vi "使用 Navigation.vi"() -> ()   [LabVIEW 2018]
uses:
  Nagivation 2.0.lvclass
panel:
  out "二维图片":picture
  out "Distance":dbl
  in  "Destination In":cluster{"X":dbl, "Y":dbl}
  in  "Source In":cluster{"X":dbl, "Y":dbl}
  out "Source Out":cluster{"X":dbl, "Y":dbl}
  out "Destination Out":cluster{"X":dbl, "Y":dbl}
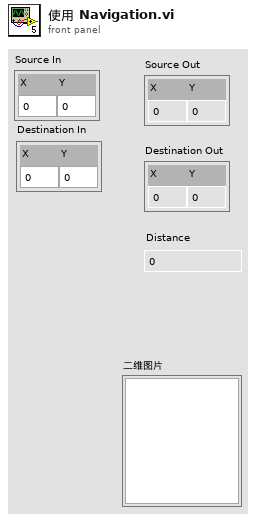
[diagram p1: front panel]
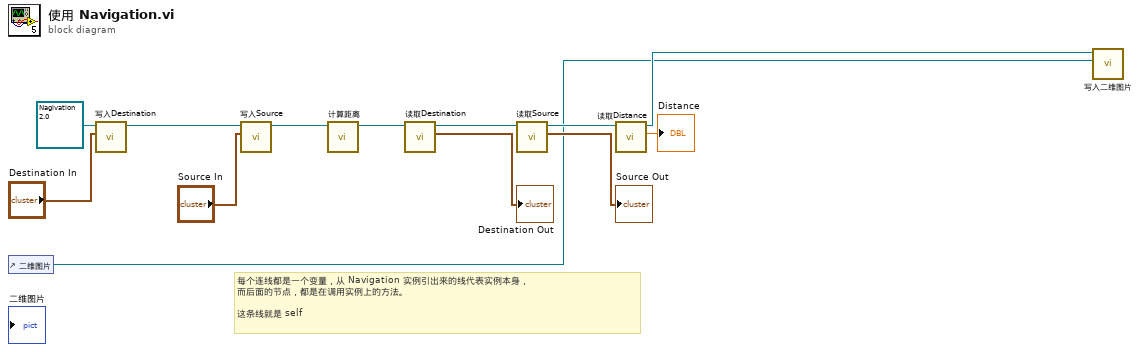
[diagram p0: block diagram]
diagram:
  # "每个连线都是一个变量，从 Navigation 实例引出来的线代表实例本身，\n而后面的节点，都是在调用实例上的方法。\n\n这条线就是 self"
  n1 = control-ref of="二维图片"() -> (w1:refnum<vi>)
  n2 = call-dynamic "写入Destination.vi"("Destination"="Destination In", "Navigation输入"=refnum<class "Nagivation 2.0.lvclass"> refnum ("Nagivation 2.0.lvclass")) -> ("Navigation输出"=w13:refnum<class "Nagivation 2.0.lvclass">)  [unwired: 8 in, 1 out]
  n3 = call-dynamic "写入Source.vi"("Source"="Source In", "Navigation输入"=w13) -> ("Navigation输出"=w7:refnum<class "Nagivation 2.0.lvclass">)  [unwired: 8 in, 1 out]
  n4 = call-dynamic "计算距离.vi"("Navigation 输入"=w7) -> ("Navigation 输出"=w6:refnum<class "Nagivation 2.0.lvclass">)  [unwired: 9 in, 1 out]
  n5 = call-dynamic "读取Destination.vi"("Navigation输入"=w6) -> ("Destination"=→"Destination Out":cluster{"X":dbl, "Y":dbl}, "Navigation输出"=w12:refnum<class "Nagivation 2.0.lvclass">)  [unwired: 8 in, 1 out]
  n6 = call-dynamic "读取Source.vi"("Navigation输入"=w12) -> ("Source"=→"Source Out":cluster{"X":dbl, "Y":dbl}, "Navigation输出"=w5:refnum<class "Nagivation 2.0.lvclass">)  [unwired: 8 in, 1 out]
  n7 = call-dynamic "读取Distance.vi"("Navigation输入"=w5) -> ("Distance"=→"Distance":dbl, "Navigation输出"=w2:refnum<class "Nagivation 2.0.lvclass">)  [unwired: 8 in, 1 out]
  n8 = call-dynamic "写入二维图片.vi"("二维图片"=w1, "Nagivation 2.0输入"=w2) -> ()  [unwired: 8 in, 2 out]
